vi "Read Channel Connection.vi"(8 "error in (no error)":errorcluster, 11 "CIF_UI in":refnum<class "CIF_UI.lvclass">) -> (0 "error out":errorcluster, 2 "Channel Connection":refnum<vi>, 3 "CIF_UI out":refnum<class "CIF_UI.lvclass">)   [LabVIEW 2021, in "CIF_UI.lvclass"]
uses:
  CIF_UI.lvclass
  CIF_UI.lvclass/CIF_UI.ctl
  Typedef/Channel Connection.ctl
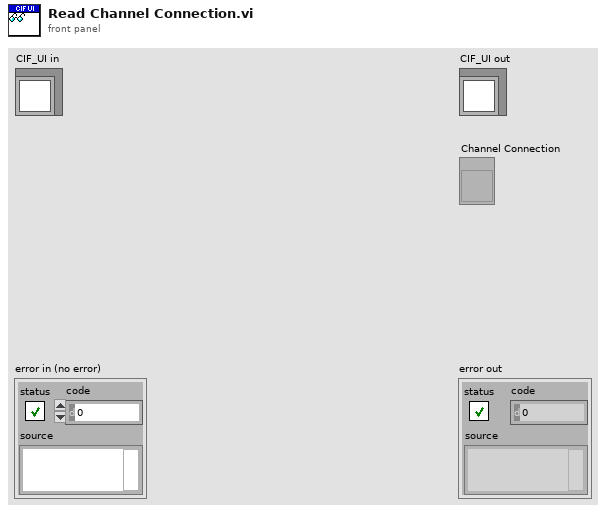
[diagram p1: front panel]
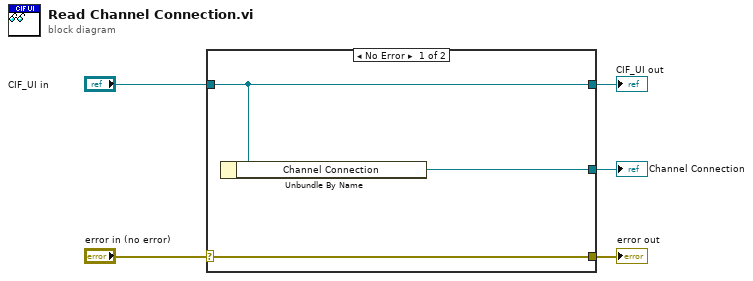
[diagram p0: block diagram]
diagram:
  n1 = case shown="No Error" "error in (no error)" {
    selector: "error in (no error)" -> [w8 w9]
    tunnel: [w8 w9] -> w4
    tunnel: [w7 w10] -> w2
    tunnel: "CIF_UI in" -> [w7 w10]
    tunnel: [w6 _] -> w1
    frame No Error {
      n2 = Unbundle By Name(w7) -> ("Channel Connection"=w6:refnum<vi>)
    }
    frame Error {
    }
  }
  "error out" <- w4
  "CIF_UI out" <- w2
  "Channel Connection" <- w1
